vi "EtherCAT Control Simplified interface.vi"() -> ()   [LabVIEW 2022 SP3]
uses:
  MOTION/TypeDefs/EL72xx_DMCOutputs.ctl
  MOTION/TypeDefs/EL72xx_DMCInputs.ctl
  SAFETY/TypeDefs/DeviceInfoData.ctl
  SAFETY/TypeDefs/FSLogicInputs.ctl
  SAFETY/TypeDefs/TwinSAFEGroupInfoData.ctl
  SAFETY/TypeDefs/TwinSAFETerminal.ctl
  IO/TypeDefs/EL2008Outputs.ctl
  <userlib>/Beckhoff-LabVIEW-Interface/_DependsOn/Base/Read/Read Sync.vi
  <userlib>/Beckhoff-LabVIEW-Interface/_DependsOn/Base/TypeResolver/Get TypeResolver.vi
  MOTION/Motion_Library.lvlib
  ADS/ADS_Library.lvlib
  SAFETY/Safety_Library.lvlib
  IO/IO_Library.lvlib
panel:
  in  "stop":bool
  in  "EtherCAT Control":T1(tab)
  in  "Move!":bool
  in  "Motion":string="<PortInfo><Inputs><SymbolControlItems><SymbolControlItem GroupName=\"ADS Write\" GroupDescription=\"Parameters for ADS Write command\"><Parameters><Parameter Name=\"Name\">Term 21 (EL7201-9014).DMC Outputs 32 Bit</Parameter><Parameter Name=\"SymbolName\">Term 21 (EL7201-9014).DMC Outputs 32 Bit</Parameter><Parameter Name=\"SymbolType\">DMC Outputs 32 Bit_1_TYPE</Parameter><Parameter Name=\"SymbolGuid\"></Parameter><Parameter Name=\"AmsNetId\">10.97.0.23.1.1</Parameter><Parameter Name=\"Port\">27911</Parameter><Parameter Name=\"IndexGroup\">#x0</Parameter><Parameter Name=\"IndexOffset\">#x0</Parameter><Parameter Name=\"BitSize\">320</Parameter><Parameter Name=\"CycleTime [ms]\">10</Parameter><Parameter Name=\"Timeout [ms]\">1000</Parameter></Parameters></SymbolControlItem></SymbolControlItems></Inputs><Outputs><SymbolControlItems><SymbolControlItem GroupName=\"ADS Read\" GroupDescription=\"Parameters for ADS Read command\"><Parameters><Parameter Name=\"Name\">Term 21 (EL7201-9014).DMC Inputs 32 Bit</Parameter><Parameter Name=\"SymbolName\">Term 21 (EL7201-9014).DMC Inputs 32 Bit</Parameter><Parameter Name=\"SymbolType\">DMC Inputs 32 Bit_1_TYPE</Parameter><Parameter Name=\"SymbolGuid\"></Parameter><Parameter Name=\"AmsNetId\">10.97.0.23.1.1</Parameter><Parameter Name=\"Port\">27911</Parameter><Parameter Name=\"IndexGroup\">#x0</Parameter><Parameter Name=\"IndexOffset\">#x0</Parameter><Parameter Name=\"BitSize\">512</Parameter><Parameter Name=\"CycleTime [ms]\">10</Parameter><Parameter Name=\"Transmode\">3</Parameter><Parameter Name=\"Timeout [ms]\">1000</Parameter><Parameter Name=\"TCBufferSize [Samples]\">10</Parameter><Parameter Name=\"LVBufferSize [Samples]\">50</Parameter><Parameter Name=\"Expected min delay [ms]\">500</Parameter></Parameters></SymbolControlItem></SymbolControlItems></Outputs></PortInfo>"
  out "bHasMatched":bool
  out "Write Status":bool
  in  "DMC Outputs":T2={"DMC"={"FeedbackControl"={"Enable latch extern on positive edge"=FALSE, "Set counter"=FALSE, "Enable latch extern on negative edge"=FALSE}, "DriveControl"={"Enable"=TRUE, "Reset"=FALSE}, "PositioningControl"={"Execute"=TRUE, "Emergency stop"=FALSE}, "Set counter value"=0, "Target position"=0, "Target velocity"=1000, "Start type"=1, "Target acceleration"=10000, "Target deceleration"=10000}}
  out "data":T3
  out "Read status?":bool
  out "error out":errorcluster
  in  "Error Ackn":bool
  out "Read status?":bool[](array[boolean])
  out "error out 2":errorcluster
  out "output cluster 3":cluster{"SymbolName":string, "Cluster":T4} {"Cluster"."Project CRC" format="%x"}
  out "output cluster 4":cluster{"SymbolName":string, "FSLogic":T5}
  out "output cluster 5":T7
  out "EL1904":T8
  out "EL2904":T8
  in  "TwinSAFE Project":string="<PortInfo><Inputs><SymbolControlItems /></Inputs><Outputs><SymbolControlItems><SymbolControlItem GroupName=\"ADS Read\" GroupDescription=\"Parameters for ADS Read command\"><Parameters><Parameter Name=\"Name\">Term 13 (EL6910).Connection Info Data</Parameter><Parameter Name=\"SymbolName\">Term 13 (EL6910).Connection Info Data</Parameter><Parameter Name=\"SymbolType\">Connection Info Data_1_TYPE</Parameter><Parameter Name=\"SymbolGuid\"></Parameter><Parameter Name=\"AmsNetId\">10.97.0.23.1.1</Parameter><Parameter Name=\"Port\">27911</Parameter><Parameter Name=\"IndexGroup\">#x0</Parameter><Parameter Name=\"IndexOffset\">#x0</Parameter><Parameter Name=\"BitSize\">48</Parameter><Parameter Name=\"CycleTime [ms]\">10</Parameter><Parameter Name=\"Transmode\">3</Parameter><Parameter Name=\"Timeout [ms]\">1000</Parameter><Parameter Name=\"TCBufferSize [Samples]\">10</Parameter><Parameter Name=\"LVBufferSize [Samples]\">50</Parameter><Parameter Name=\"Expected min delay [ms]\">500</Parameter></Parameters></SymbolControlItem><SymbolControlItem GroupName=\"ADS Read\" GroupDescription=\"Parameters for ADS Read command\"><Parameters><Parameter Name=\"Name\">Term 13 (EL6910).Device Info Data</Parameter><Parameter Name=\"SymbolName\">Term 13 (EL6910).Device Info Data</Parameter><Parameter Name=\"SymbolType\">Device Info Data_1_TYPE</Parameter><Parameter Name=\"SymbolGuid\"></Parameter><Parameter Name=\"AmsNetId\">10.97.0.23.1.1</Parameter><Parameter Name=\"Port\">27911</Parameter><Parameter Name=\"IndexGroup\">#x0</Parameter><Parameter Name=\"IndexOffset\">#x0</Parameter><Parameter Name=\"BitSize\">48</Parameter><Parameter Name=\"CycleTime [ms]\">10</Parameter><Parameter Name=\"Transmode\">3</Parameter><Parameter Name=\"Timeout [ms]\">1000</Parameter><Parameter Name=\"TCBufferSize [Samples]\">10</Parameter><Parameter Name=\"LVBufferSize [Samples]\">50</Parameter><Parameter Name=\"Expected min delay [ms]\">500</Parameter></Parameters></SymbolControlItem><SymbolControlItem GroupName=\"ADS Read\" GroupDescription=\"Parameters for ADS Read command\"><Parameters><Parameter Name=\"Name\">Term 13 (EL6910).FSLOGIC Inputs</Parameter><Parameter Name=\"SymbolName\">Term 13 (EL6910).FSLOGIC Inputs</Parameter><Parameter Name=\"SymbolType\">FSLOGIC Inputs_1_TYPE</Parameter><Parameter Name=\"SymbolGuid\"></Parameter><Parameter Name=\"AmsNetId\">10.97.0.23.1.1</Parameter><Parameter Name=\"Port\">27911</Parameter><Parameter Name=\"IndexGroup\">#x0</Parameter><Parameter Name=\"IndexOffset\">#x0</Parameter><Parameter Name=\"BitSize\">16</Parameter><Parameter Name=\"CycleTime [ms]\">10</Parameter><Parameter Name=\"Transmode\">3</Parameter><Parameter Name=\"Timeout [ms]\">1000</Parameter><Parameter Name=\"TCBufferSize [Samples]\">10</Parameter><Parameter Name=\"LVBufferSize [Samples]\">50</Parameter><Parameter Name=\"Expected min delay [ms]\">500</Parameter></Parameters></SymbolControlItem><SymbolControlItem GroupName=\"ADS Read\" GroupDescription=\"Parameters for ADS Read command\"><Parameters><Parameter Name=\"Name\">Term 13 (EL6910).TwinSAFE Group Info Data.TwinSafeGroup1 Info Data</Parameter><Parameter Name=\"SymbolName\">Term 13 (EL6910).TwinSAFE Group Info Data.TwinSafeGroup1 Info Data</Parameter><Parameter Name=\"SymbolType\">INFODATA_GRP_3</Parameter><Parameter Name=\"SymbolGuid\"></Parameter><Parameter Name=\"AmsNetId\">10.97.0.23.1.1</Parameter><Parameter Name=\"Port\">27911</Parameter><Parameter Name=\"IndexGroup\">#x0</Parameter><Parameter Name=\"IndexOffset\">#x0</Parameter><Parameter Name=\"BitSize\">16</Parameter><Parameter Name=\"CycleTime [ms]\">10</Parameter><Parameter Name=\"Transmode\">3</Parameter><Parameter Name=\"Timeout [ms]\">1000</Parameter><Parameter Name=\"TCBufferSize [Samples]\">10</Parameter><Parameter Name=\"LVBufferSize [Samples]\">50</Parameter><Parameter Name=\"Expected min delay [ms]\">500</Parameter></Parameters></SymbolControlItem></SymbolControlItems></Outputs></PortInfo>"
  in  "PLC Safety Control":string="<PortInfo><Inputs><SymbolControlItems><SymbolControlItem GroupName=\"ADS Write\" GroupDescription=\"Parameters for ADS Write command\"><Parameters><Parameter Name=\"Name\">MAIN.SafetyErrAck</Parameter><Parameter Name=\"SymbolName\">MAIN.SafetyErrAck</Parameter><Parameter Name=\"SymbolType\">BOOL</Parameter><Parameter Name=\"SymbolGuid\"></Parameter><Parameter Name=\"AmsNetId\">10.97.0.23.1.1</Parameter><Parameter Name=\"Port\">851</Parameter><Parameter Name=\"IndexGroup\">#x0</Parameter><Parameter Name=\"IndexOffset\">#x0</Parameter><Parameter Name=\"BitSize\">8</Parameter><Parameter Name=\"CycleTime [ms]\">10</Parameter><Parameter Name=\"Timeout [ms]\">1000</Parameter></Parameters></SymbolControlItem></SymbolControlItems></Inputs><Outputs><SymbolControlItems /></Outputs></PortInfo>"
  out "Write Status":bool
  out "bHasMatched":bool
  out "error out 5":errorcluster
  in  "Digital Outputs":string="<PortInfo><Inputs><SymbolControlItems><SymbolControlItem GroupName=\"ADS Write\" GroupDescription=\"Parameters for ADS Write command\"><Parameters><Parameter Name=\"Name\">Term 2 (EL2008).Channel 1.Output</Parameter><Parameter Name=\"SymbolName\">Term 2 (EL2008).Channel 1.Output</Parameter><Parameter Name=\"SymbolType\">BIT</Parameter><Parameter Name=\"SymbolGuid\"></Parameter><Parameter Name=\"AmsNetId\">10.97.0.23.1.1</Parameter><Parameter Name=\"Port\">27905</Parameter><Parameter Name=\"IndexGroup\">#x0</Parameter><Parameter Name=\"IndexOffset\">#x0</Parameter><Parameter Name=\"BitSize\">1</Parameter><Parameter Name=\"CycleTime [ms]\">2</Parameter><Parameter Name=\"Timeout [ms]\">1000</Parameter></Parameters></SymbolControlItem><SymbolControlItem GroupName=\"ADS Write\" GroupDescription=\"Parameters for ADS Write command\"><Parameters><Parameter Name=\"Name\">Term 2 (EL2008).Channel 2.Output</Parameter><Parameter Name=\"SymbolName\">Term 2 (EL2008).Channel 2.Output</Parameter><Parameter Name=\"SymbolType\">BIT</Parameter><Parameter Name=\"SymbolGuid\"></Parameter><Parameter Name=\"AmsNetId\">10.97.0.23.1.1</Parameter><Parameter Name=\"Port\">27905</Parameter><Parameter Name=\"IndexGroup\">#x0</Parameter><Parameter Name=\"IndexOffset\">#x0</Parameter><Parameter Name=\"BitSize\">1</Parameter><Parameter Name=\"CycleTime [ms]\">2</Parameter><Parameter Name=\"Timeout [ms]\">1000</Parameter></Parameters></SymbolControlItem><SymbolControlItem GroupName=\"ADS Write\" GroupDescription=\"Parameters for ADS Write command\"><Parameters><Parameter Name=\"Name\">Term 2 (EL2008).Channel 3.Output</Parameter><Parameter Name=\"SymbolName\">Term 2 (EL2008).Channel 3.Output</Parameter><Parameter Name=\"SymbolType\">BIT</Parameter><Parameter Name=\"SymbolGuid\"></Parameter><Parameter Name=\"AmsNetId\">10.97.0.23.1.1</Parameter><Parameter Name=\"Port\">27905</Parameter><Parameter Name=\"IndexGroup\">#x0</Parameter><Parameter Name=\"IndexOffset\">#x0</Parameter><Parameter Name=\"BitSize\">1</Parameter><Parameter Name=\"CycleTime [ms]\">2</Parameter><Parameter Name=\"Timeout [ms]\">1000</Parameter></Parameters></SymbolControlItem><SymbolControlItem GroupName=\"ADS Write\" GroupDescription=\"Parameters for ADS Write command\"><Parameters><Parameter Name=\"Name\">Term 2 (EL2008).Channel 4.Output</Parameter><Parameter Name=\"SymbolName\">Term 2 (EL2008).Channel 4.Output</Parameter><Parameter Name=\"SymbolType\">BIT</Parameter><Parameter Name=\"SymbolGuid\"></Parameter><Parameter Name=\"AmsNetId\">10.97.0.23.1.1</Parameter><Parameter Name=\"Port\">27905</Parameter><Parameter Name=\"IndexGroup\">#x0</Parameter><Parameter Name=\"IndexOffset\">#x0</Parameter><Parameter Name=\"BitSize\">1</Parameter><Parameter Name=\"CycleTime [ms]\">2</Parameter><Parameter Name=\"Timeout [ms]\">1000</Parameter></Parameters></SymbolControlItem><SymbolControlItem GroupName=\"ADS Write\" GroupDescription=\"Parameters for ADS Write command\"><Parameters><Parameter Name=\"Name\">Term 2 (EL2008).Channel 5.Output</Parameter><Parameter Name=\"SymbolName\">Term 2 (EL2008).Channel 5.Output</Parameter><Parameter Name=\"SymbolType\">BIT</Parameter><Parameter Name=\"SymbolGuid\"></Parameter><Parameter Name=\"AmsNetId\">10.97.0.23.1.1</Parameter><Parameter Name=\"Port\">27905</Parameter><Parameter Name=\"IndexGroup\">#x0</Parameter><Parameter Name=\"IndexOffset\">#x0</Parameter><Parameter Name=\"BitSize\">1</Parameter><Parameter Name=\"CycleTime [ms]\">2</Parameter><Parameter Name=\"Timeout [ms]\">1000</Parameter></Parameters></SymbolControlItem><SymbolControlItem GroupName=\"ADS Write\" GroupDescription=\"Parameters for ADS Write command\"><Parameters><Parameter Name=\"Name\">Term 2 (EL2008).Channel 6.Output</Parameter><Parameter Name=\"SymbolName\">Term 2 (EL2008).Channel 6.Output</Parameter><Parameter Name=\"SymbolType\">BIT</Parameter><Parameter Name=\"SymbolGuid\"></Parameter><Parameter Name=\"AmsNetId\">10.97.0.23.1.1</Parameter><Parameter Name=\"Port\">27905</Parameter><Parameter Name=\"IndexGroup\">#x0</Parameter><Parameter Name=\"IndexOffset\">#x0</Parameter><Parameter Name=\"BitSize\">1</Parameter><Parameter Name=\"CycleTime [ms]\">2</Parameter><Parameter Name=\"Timeout [ms]\">1000</Parameter></Parameters></SymbolControlItem><SymbolControlItem GroupName=\"ADS Write\" GroupDescription=\"Parameters for ADS Write command\"><Parameters><Parameter Name=\"Name\">Term 2 (EL2008).Channel 7.Output</Parameter><Parameter Name=\"SymbolName\">Term 2 (EL2008).Channel 7.Output</Parameter><Parameter Name=\"SymbolType\">BIT</Parameter><Parameter Name=\"SymbolGuid\"></Parameter><Parameter Name=\"AmsNetId\">10.97.0.23.1.1</Parameter><Parameter Name=\"Port\">27905</Parameter><Parameter Name=\"IndexGroup\">#x0</Parameter><Parameter Name=\"IndexOffset\">#x0</Parameter><Parameter Name=\"BitSize\">1</Parameter><Parameter Name=\"CycleTime [ms]\">2</Parameter><Parameter Name=\"Timeout [ms]\">1000</Parameter></Parameters></SymbolControlItem><SymbolControlItem GroupName=\"ADS Write\" GroupDescription=\"Parameters for ADS Write command\"><Parameters><Parameter Name=\"Name\">Term 2 (EL2008).Channel 8.Output</Parameter><Parameter Name=\"SymbolName\">Term 2 (EL2008).Channel 8.Output</Parameter><Parameter Name=\"SymbolType\">BIT</Parameter><Parameter Name=\"SymbolGuid\"></Parameter><Parameter Name=\"AmsNetId\">10.97.0.23.1.1</Parameter><Parameter Name=\"Port\">27905</Parameter><Parameter Name=\"IndexGroup\">#x0</Parameter><Parameter Name=\"IndexOffset\">#x0</Parameter><Parameter Name=\"BitSize\">1</Parameter><Parameter Name=\"CycleTime [ms]\">2</Parameter><Parameter Name=\"Timeout [ms]\">1000</Parameter></Parameters></SymbolControlItem></SymbolControlItems></Inputs><Outputs><SymbolControlItems /></Outputs></PortInfo>"
  out "bHasMatched":bool[](array[boolean])
  out "Write Status":bool[](array[boolean])
  in  "EL2008 Channels":T9
  out "error out 3":errorcluster
  in  "Digital Outputs":string="<PortInfo><Inputs><SymbolControlItems><SymbolControlItem GroupName=\"ADS Write\" GroupDescription=\"Parameters for ADS Write command\"><Parameters><Parameter Name=\"Name\">Box 17 (NI 9145).Module 1 (NI 9472).Digital Output.DO</Parameter><Parameter Name=\"SymbolName\">Box 17 (NI 9145).Module 1 (NI 9472).Digital Output.DO</Parameter><Parameter Name=\"SymbolType\">USINT</Parameter><Parameter Name=\"SymbolGuid\"></Parameter><Parameter Name=\"AmsNetId\">10.97.0.23.1.1</Parameter><Parameter Name=\"Port\">27911</Parameter><Parameter Name=\"IndexGroup\">#x0</Parameter><Parameter Name=\"IndexOffset\">#x0</Parameter><Parameter Name=\"BitSize\">8</Parameter><Parameter Name=\"CycleTime [ms]\">10</Parameter><Parameter Name=\"Timeout [ms]\">1000</Parameter></Parameters></SymbolControlItem></SymbolControlItems></Inputs><Outputs><SymbolControlItems /></Outputs></PortInfo>"
  out "error out":errorcluster
  out "bHasMatched":bool
  out "Write Status":bool
  in  "NI9472":T9
  out "Waveform Chart 2":dbl(graph)
  out "RData":variant
  out "RDataArray":variant[](array[variant])
  out "Read status? 3":bool
  in  "String":string="<PortInfo><Inputs><SymbolControlItems /></Inputs><Outputs><SymbolControlItems><SymbolControlItem GroupName=\"ADS Read\" GroupDescription=\"Parameters for ADS Read command\"><Parameters><Parameter Name=\"Name\">Term 15 (EL3255).AI Standard Channel 1.Value</Parameter><Parameter Name=\"SymbolName\">Term 15 (EL3255).AI Standard Channel 1.Value</Parameter><Parameter Name=\"SymbolType\">INT</Parameter><Parameter Name=\"SymbolGuid\"></Parameter><Parameter Name=\"AmsNetId\">10.97.0.23.1.1</Parameter><Parameter Name=\"Port\">27911</Parameter><Parameter Name=\"IndexGroup\">#x0</Parameter><Parameter Name=\"IndexOffset\">#x0</Parameter><Parameter Name=\"BitSize\">16</Parameter><Parameter Name=\"CycleTime [ms]\">10</Parameter><Parameter Name=\"Transmode\">3</Parameter><Parameter Name=\"Timeout [ms]\">1000</Parameter><Parameter Name=\"TCBufferSize [Samples]\">10</Parameter><Parameter Name=\"LVBufferSize [Samples]\">50</Parameter><Parameter Name=\"Expected min delay [ms]\">500</Parameter></Parameters></SymbolControlItem></SymbolControlItems></Outputs></PortInfo>"
  out "error out 4":errorcluster
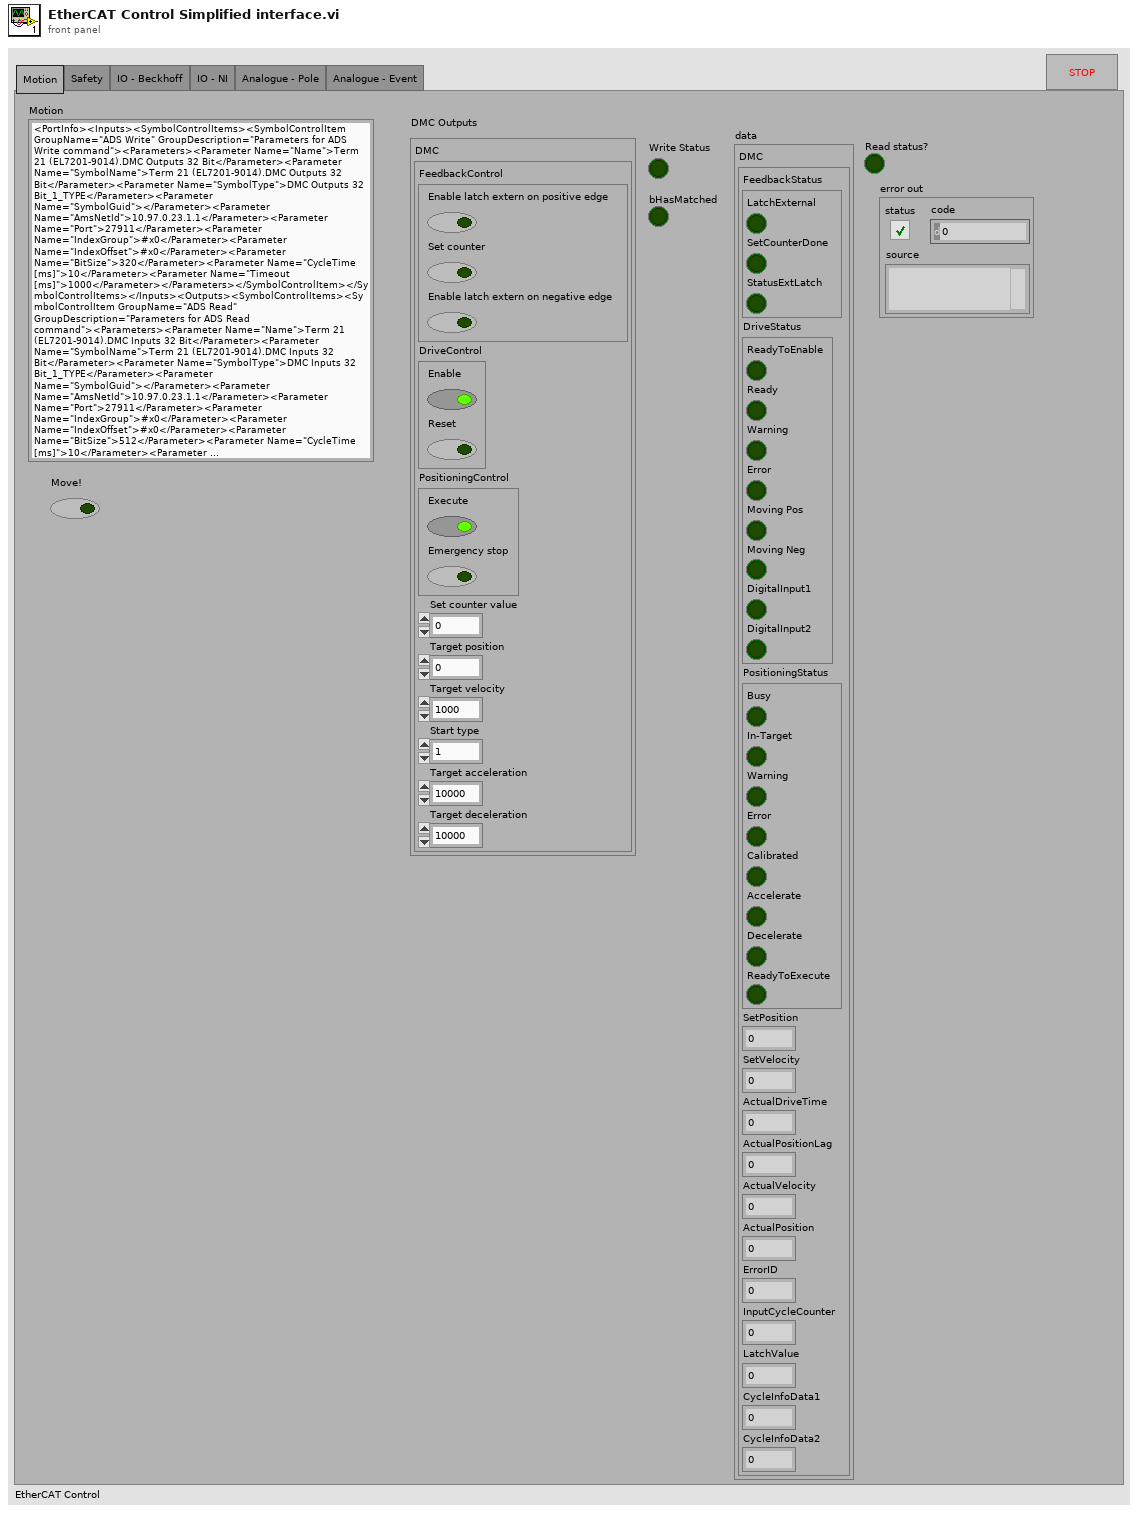
[diagram p1: front panel]
types:
  T1 = enum32{"Motion", "Safety", "IO - Beckhoff", "IO - NI", "Analogue - Pole", "Analogue - Event"}
  T2 = typedef "Motion_Library.lvlib/EL72xx_DMCOutputs.ctl" = cluster{"DMC":cluster{"FeedbackControl":cluster{"Enable latch extern on positive edge":bool, "Set counter":bool, "Enable latch extern on negative edge":bool}, "DriveControl":cluster{"Enable":bool, "Reset":bool}, "PositioningControl":cluster{"Execute":bool, "Emergency stop":bool}, "Set counter value":i32, "Target position":i32, "Target velocity":i16, "Start type":u16, "Target acceleration":u16, "Target deceleration":u16}}
  T3 = typedef "Motion_Library.lvlib/EL72xx_DMCInputs.ctl" = cluster{"DMC":cluster{"FeedbackStatus":cluster{"LatchExternal":bool, "SetCounterDone":bool, "StatusExtLatch":bool}, "DriveStatus":cluster{"ReadyToEnable":bool, "Ready":bool, "Warning":bool, "Error":bool, "Moving Pos":bool, "Moving Neg":bool, "DigitalInput1":bool, "DigitalInput2":bool}, "PositioningStatus":cluster{"Busy":bool, "In-Target":bool, "Warning":bool, "Error":bool, "Calibrated":bool, "Accelerate":bool, "Decelerate":bool, "ReadyToExecute":bool}, "SetPosition":dbl, "SetVelocity":dbl, "ActualDriveTime":dbl, "ActualPositionLag":dbl, "ActualVelocity":dbl, "ActualPosition":dbl, "ErrorID":dbl, "InputCycleCounter":dbl, "LatchValue":dbl, "CycleInfoData1":dbl, "CycleInfoData2":dbl}}
  T4 = typedef "Safety_Library.lvlib/DeviceInfoData.ctl" = cluster{"Project CRC":u16, "Serial Number":u32}
  T5 = typedef "Safety_Library.lvlib/FSLogicInputs.ctl" = cluster{"Safe Logic State":u8, "Cycle Counter":u8}
  T6 = typedef "Safety_Library.lvlib/TwinSAFEGroupInfoData.ctl" = cluster{"State":u8, "Diag":u8}
  T7 = cluster{"SymbolName":string, "Group Info Data":T6}
  T8 = typedef "Safety_Library.lvlib/TwinSAFETerminal.ctl" = cluster{"SymbolName":string, "State":dbl, "Diag":dbl, "Channel 1":bool, "Channel 2":bool, "Channel 3":bool, "Channel 4":bool}
  T9 = typedef "IO_Library.lvlib/EL2008Outputs.ctl" = cluster{"Channel 1":bool, "Channel 2":bool, "Channel 3":bool, "Channel 4":bool, "Channel 5":bool, "Channel 6":bool, "Channel 7":bool, "Channel 8":bool}
  T10 = cluster{"State":dbl, "State 2":dbl, "State 3":i8}
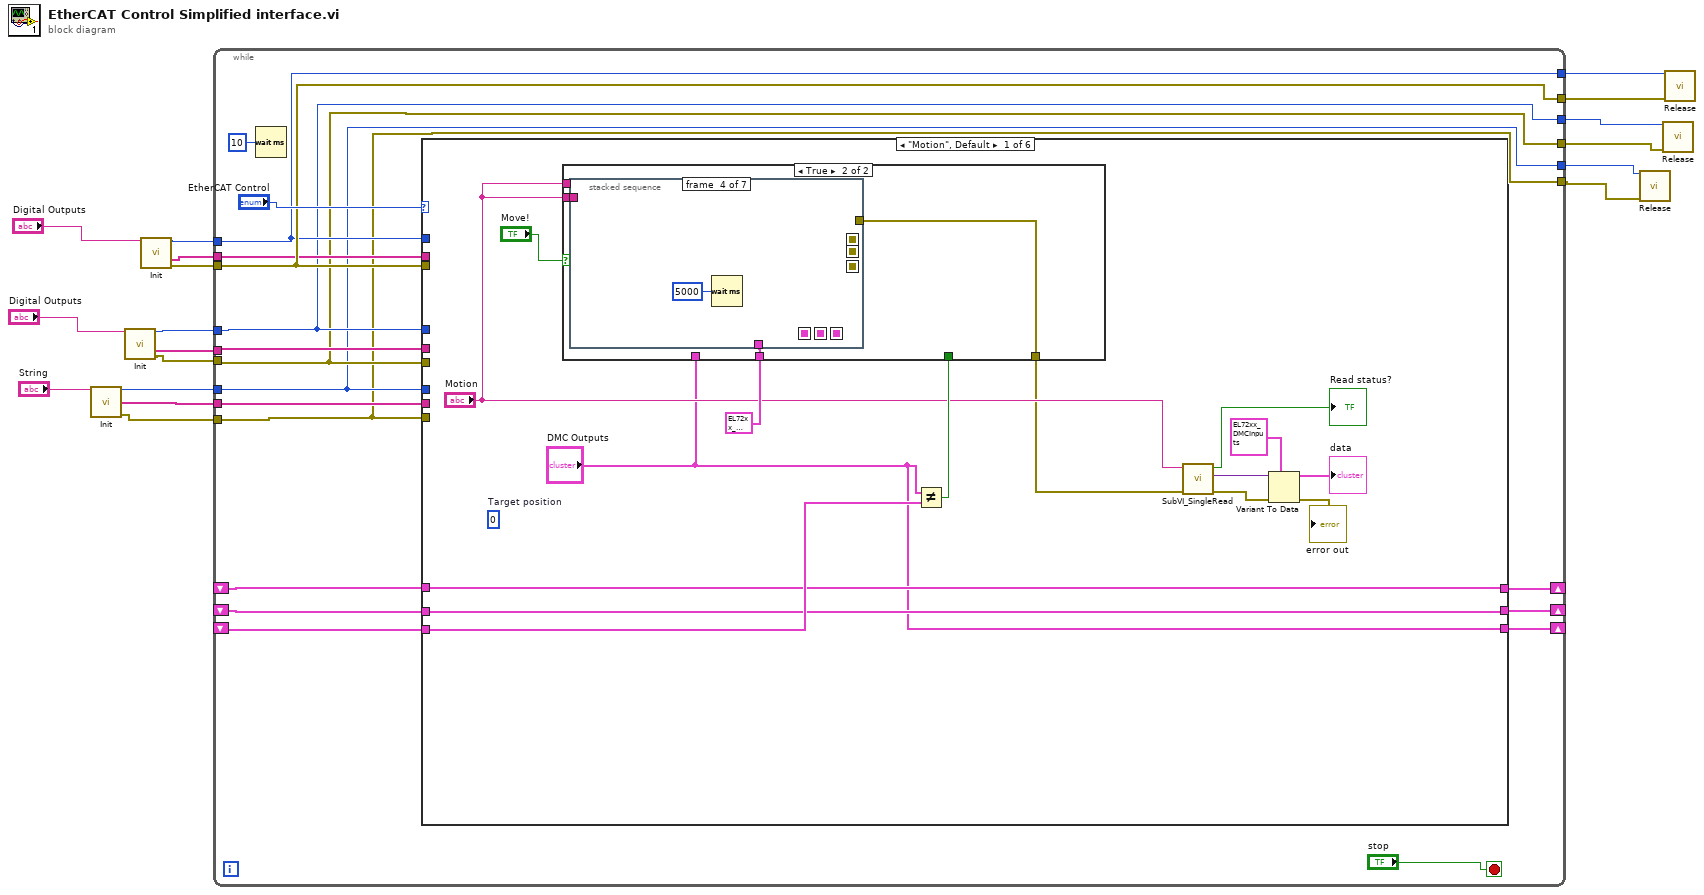
[diagram p0: block diagram]
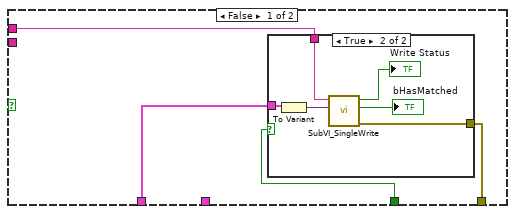
[diagram p2: hidden frame]
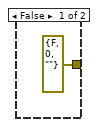
[diagram p3: hidden frame]
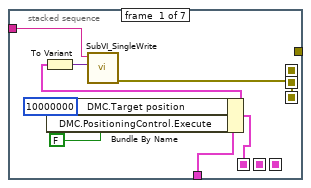
[diagram p4: hidden frame]
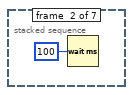
[diagram p5: hidden frame]
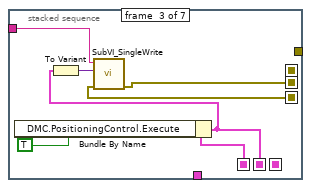
[diagram p6: hidden frame]
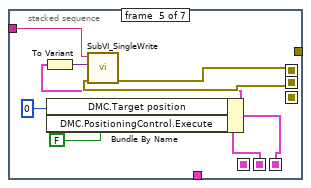
[diagram p7: hidden frame]
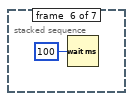
[diagram p8: hidden frame]
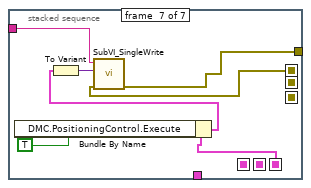
[diagram p9: hidden frame]
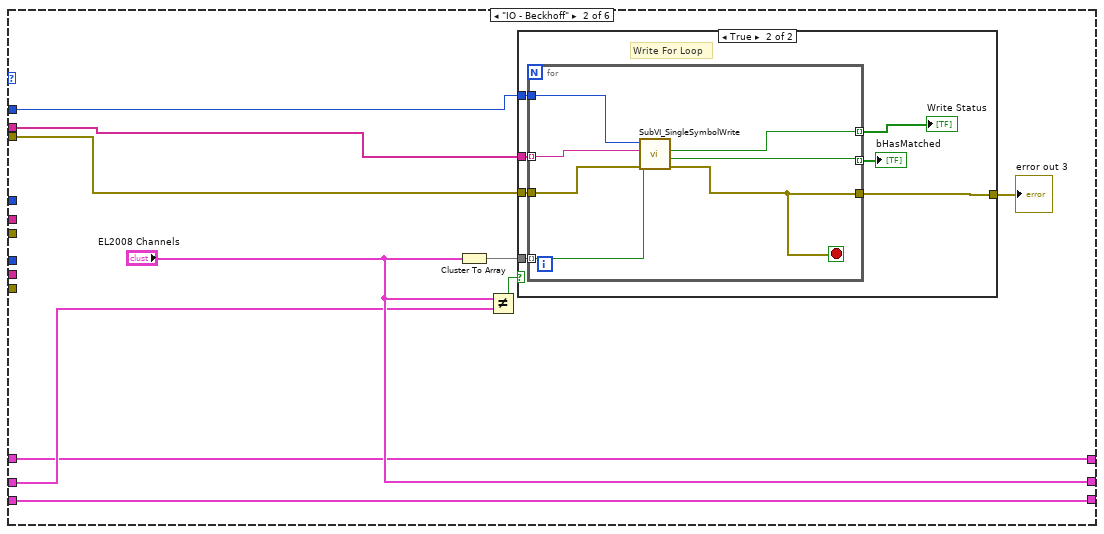
[diagram p10: hidden frame]
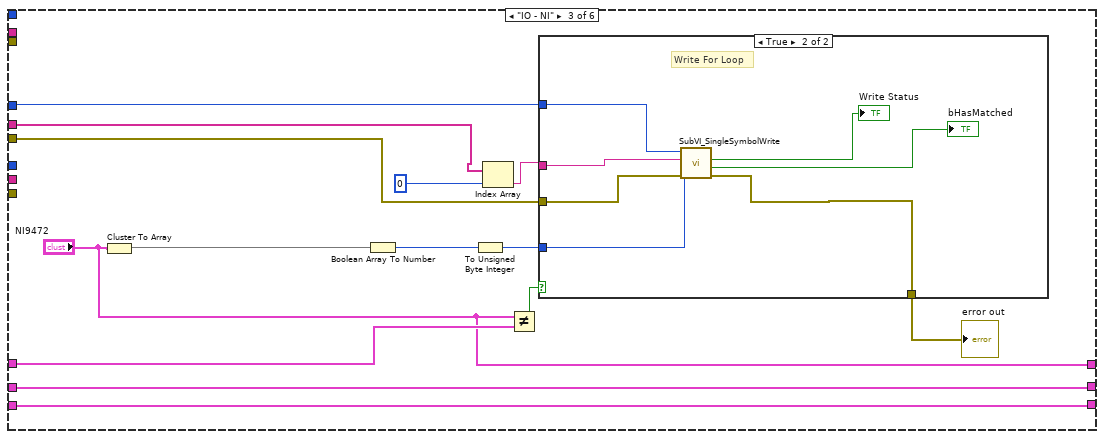
[diagram p12: hidden frame]
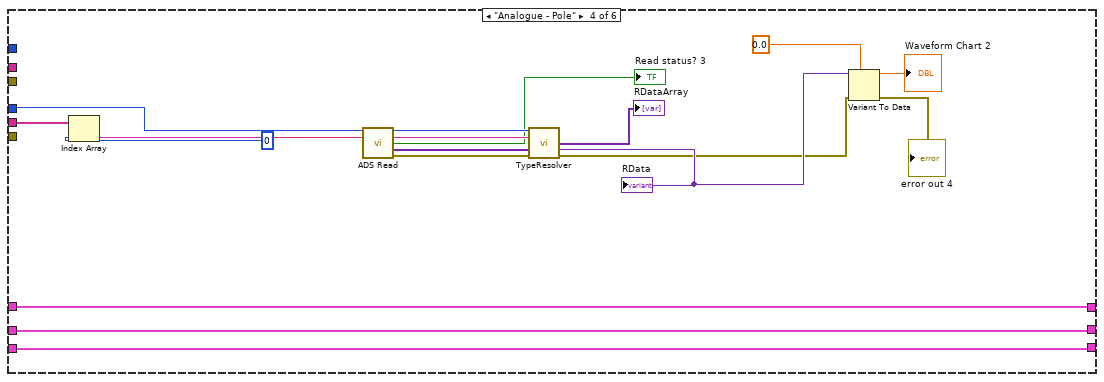
[diagram p14: hidden frame]
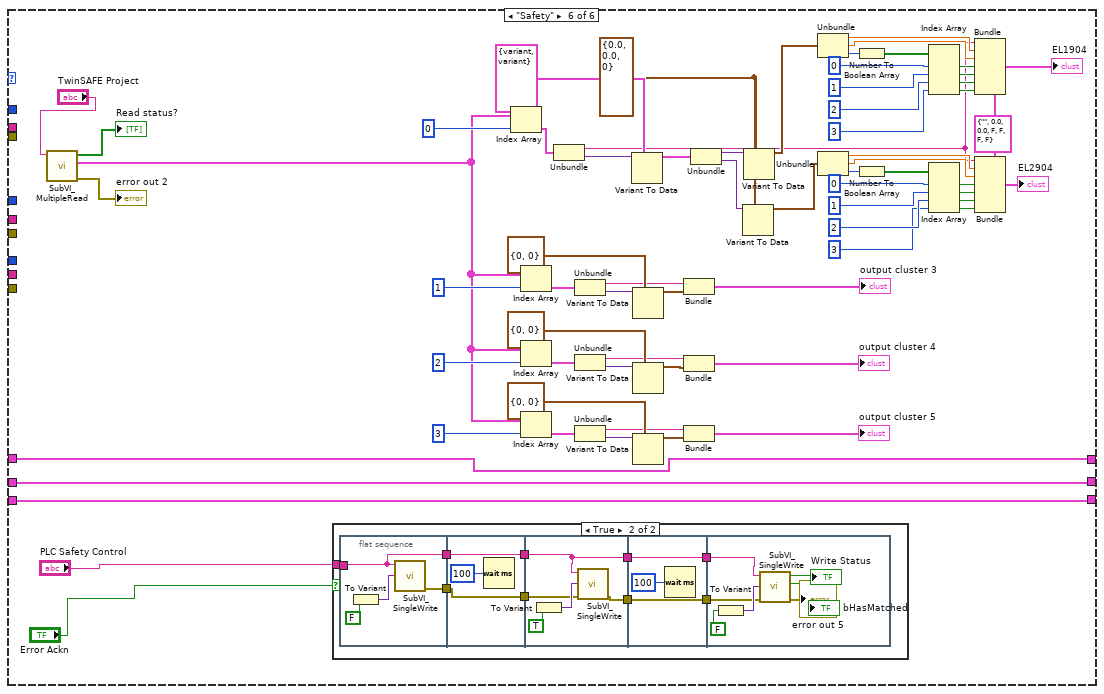
[diagram p16: hidden frame]
diagram:
  n1 = call <userlib>:"Init.vi"("XMLDescription"="String") -> ("Handle"=w5:u32, "ReadGrpSymbols"=w4:string[], "error out"=w3:errorcluster)  [unwired: 10 in, 2 out]
  n2 = call <userlib>:"Init.vi"("XMLDescription"="Digital Outputs") -> ("Handle"=w11:u32, "WriteGrpSymbols"=w10:string[], "error out"=w9:errorcluster)  [unwired: 10 in, 2 out]
  n3 = call <userlib>:"Init.vi"("XMLDescription"="Digital Outputs") -> ("Handle"=w16:u32, "WriteGrpSymbols"=w13:string[], "error out"=w15:errorcluster)  [unwired: 10 in, 2 out]
  n4 = while {
    shift-right: [w32] -> _
    shift-left: _ -> [w33]
    tunnel: [w28] -> w17
    tunnel: w16 -> [w28]
    tunnel: w15 -> [w29]
    tunnel: [w29] -> w14
    shift-right: [w31] -> _
    shift-left: _ -> [w30]
    tunnel: w13 -> [w27]
    tunnel: w11 -> [w25]
    tunnel: w10 -> [w26]
    tunnel: w9 -> [w24]
    tunnel: [w25] -> w8
    tunnel: [w24] -> w7
    shift-right: [w23] -> _
    shift-left: _ -> [w22]
    tunnel: w5 -> [w20]
    tunnel: w4 -> [w21]
    tunnel: w3 -> [w19]
    tunnel: [w20] -> w2
    tunnel: [w19] -> w1
    stop <- "stop" stop-if-true
    n5 = Wait (ms)(milliseconds to wait=u32 10) -> ()  [unwired: 1 out]
    n6 = case shown="\"Motion\", Default" "EtherCAT Control" {
      tunnel: w33 -> [w45 w107 w136 w162 w165 w233]
      tunnel: ["DMC Outputs" w107 w136 w162 w165 w233] -> w32
      tunnel: [w44 "EL2008 Channels" w135 w161 w164 w169] -> w31
      tunnel: w30 -> [w44 w101 w135 w161 w164 w169]
      tunnel: w29 -> [_ w105 _ _ _ _]
      tunnel: w28 -> [_ w104 _ _ _ _]
      tunnel: w27 -> [_ w103 _ _ _ _]
      tunnel: w25 -> [_ _ w134 _ _ _]
      tunnel: w26 -> [_ _ w124 _ _ _]
      tunnel: w24 -> [_ _ w133 _ _ _]
      tunnel: [w43 w98 "NI9472" w160 w163 w168] -> w23
      tunnel: w22 -> [w43 w98 w132 w160 w163 w168]
      tunnel: w20 -> [_ _ _ w146 _ _]
      tunnel: w21 -> [_ _ _ w147 _ _]
      tunnel: w19 -> [_ _ _ _ _ _]
      frame "Motion", Default {
        (unwired) 0  # Target position
        n7 = Not Equal?(x="DMC Outputs", y=w45) -> (x != y?=w40:bool)
        n8 = case shown="True" "Move!" {
          tunnel: "Motion" -> [_ w65]
          tunnel: T2 {"DMC"={"FeedbackControl"={"Enable latch extern on positive edge"=FALSE, "Set counter"=FALSE, "Enable latch extern on negative edge"=FALSE}, "DriveControl"={"Enable"=TRUE, "Reset"=FALSE}, "PositioningControl"={"Execute"=TRUE, "Emergency stop"=FALSE}, "Set counter value"=0, "Target position"=0, "Target velocity"=1000, "Start type"=1, "Target acceleration"=10000, "Target deceleration"=10000}} ("DMC Outputs") -> [_ w64]
          tunnel: w40 -> [w55 _]
          tunnel: "Motion" -> [w54 _]
          tunnel: "DMC Outputs" -> [w53 _]
          tunnel: [w52 w63] -> w37
          frame False {
            n9 = case shown="True" w55 {
              tunnel: w54 -> [_ w62]
              tunnel: [errorcluster {"status"=FALSE, "code"=0, "source"=""} ("error out") w60] -> w52
              tunnel: w53 -> [_ w57]
              frame False {
              }
              frame True {
                n10 = To Variant(anything=w57) -> (Variant=w61:variant)
                n11 = call "SubVI_SingleWrite.vi"("WData"=w61, "String"=w62) -> ("error out"=w60:errorcluster, "bHasMatched"=→"bHasMatched":bool, "Write Status"=→"Write Status":bool)  [unwired: 6 in, 1 out]
              }
            }
          }
          frame True {
            n12 = stacked-sequence {
              seq-local: [w68 _ _ _ _ _ _] -> [_ _ w78 _ _ _ _]
              seq-local: [_ _ w76 _ _ _ _] -> [_ _ _ _ w85 _ _]
              seq-local: [_ _ _ _ w84 _ _] -> [_ _ _ _ _ _ w93]
              seq-local: [w66 _ _ _ _ _ _] -> [_ _ w75 _ _ _ _]
              seq-local: [_ _ w74 _ _ _ _] -> [_ _ _ _ w83 _ _]
              seq-local: [_ _ _ _ w82 _ _] -> [_ _ _ _ _ _ w91]
              tunnel: w65 -> [w67 _ w77 _ w86 _ w94]
              tunnel: w64 -> [w71 _ _ _ _ _ _]
              tunnel: [_ _ _ _ _ _ w92] -> w63
              frame #0 {
                n13 = Bundle By Name(cluster=w71, "DMC.Target position"=10000000, "DMC.PositioningControl.Execute"=FALSE ("DMC.DriveControl.Reset")) -> (w66:T2)
                n14 = To Variant(anything=w66) -> (Variant=w72:variant)
                n15 = call "SubVI_SingleWrite.vi"("WData"=w72, "String"=w67) -> ("error out"=w68:errorcluster)  [unwired: 6 in, 3 out]
              }
              frame #1 {
                n16 = Wait (ms)(milliseconds to wait=u32 100) -> ()  [unwired: 1 out]
              }
              frame #2 {
                n17 = Bundle By Name(cluster=w75, "DMC.PositioningControl.Execute"=TRUE ("DMC.DriveControl.Reset")) -> (w74:T2)
                n18 = To Variant(anything=w74) -> (Variant=w79:variant)
                n19 = call "SubVI_SingleWrite.vi"("error in"=w78, "WData"=w79, "String"=w77) -> ("error out"=w76:errorcluster)  [unwired: 5 in, 3 out]
              }
              frame #3 {
                n20 = Wait (ms)(milliseconds to wait=u32 5000) -> ()  [unwired: 1 out]
              }
              frame #4 {
                n21 = Bundle By Name(cluster=w83, "DMC.Target position"=0, "DMC.PositioningControl.Execute"=FALSE ("DMC.DriveControl.Reset")) -> (w82:T2)
                n22 = To Variant(anything=w82) -> (Variant=w89:variant)
                n23 = call "SubVI_SingleWrite.vi"("error in"=w85, "WData"=w89, "String"=w86) -> ("error out"=w84:errorcluster)  [unwired: 5 in, 3 out]
              }
              frame #5 {
                n24 = Wait (ms)(milliseconds to wait=u32 100) -> ()  [unwired: 1 out]
              }
              frame #6 {
                n25 = Bundle By Name(cluster=w91, "DMC.PositioningControl.Execute"=TRUE ("DMC.DriveControl.Reset")) -> (w95:T2)
                n26 = To Variant(anything=w95) -> (Variant=w96:variant)
                n27 = call "SubVI_SingleWrite.vi"("error in"=w93, "WData"=w96, "String"=w94) -> ("error out"=w92:errorcluster)  [unwired: 5 in, 3 out]
              }
            }
          }
        }
        n28 = call "SubVI_SingleRead.vi"("error in"=w37, "String"="Motion") -> ("error out"=w49:errorcluster, "RData"=w50:variant, "Read status?"=→"Read status?":bool)  [unwired: 6 in]
        n29 = Variant To Data(error in=w49, type=T3 {"DMC"={"FeedbackStatus"={"LatchExternal"=FALSE, "SetCounterDone"=FALSE, "StatusExtLatch"=FALSE}, "DriveStatus"={"ReadyToEnable"=FALSE, "Ready"=FALSE, "Warning"=FALSE, "Error"=FALSE, "Moving Pos"=FALSE, "Moving Neg"=FALSE, "DigitalInput1"=FALSE, "DigitalInput2"=FALSE}, "PositioningStatus"={"Busy"=FALSE, "In-Target"=FALSE, "Warning"=FALSE, "Error"=FALSE, "Calibrated"=FALSE, "Accelerate"=FALSE, "Decelerate"=FALSE, "ReadyToExecute"=FALSE}, "SetPosition"=0.0, "SetVelocity"=0.0, "ActualDriveTime"=0.0, "ActualPositionLag"=0.0, "ActualVelocity"=0.0, "ActualPosition"=0.0, "ErrorID"=0.0, "InputCycleCounter"=0.0, "LatchValue"=0.0, "CycleInfoData1"=0.0, "CycleInfoData2"=0.0}} ("DMC Inputs"), Variant=w50) -> (data=→"data":T3, error out=→"error out":errorcluster)
      }
      frame "IO - Beckhoff" {
        n30 = Cluster To Array(cluster="EL2008 Channels") -> (array=w106:bool[])
        n31 = Not Equal?(x="EL2008 Channels", y=w101) -> (x != y?=w100:bool)
        n32 = case shown="True" w100 {
          tunnel: w106 -> [_ w113]
          tunnel: w105 -> [w108 w112]
          tunnel: w104 -> [_ w111]
          tunnel: w103 -> [_ w110]
          tunnel: [w108 w109] -> w99
          frame False {
          }
          frame True {
            # "Write For Loop"
            n33 = for {
              tunnel: w110 -> [w121] mode=indexing
              tunnel: w112 -> [w120]
              tunnel: w111 -> [w122]
              tunnel: [w118] -> w114 mode=indexing
              tunnel: [w119] -> w115 mode=indexing
              tunnel: w113 -> [w117] mode=indexing
              tunnel: [w116] -> w109
              stop <- w116 stop-if-true
              n34 = call "SubVI_SingleSymbolWrite.vi"("error in"=w120, "WData"=w117, "SymbolName"=w121, "Handle In"=w122) -> ("error out"=w116:errorcluster, "bHasMatched"=w118:bool, "Write Status"=w119:bool)  [unwired: 4 in, 1 out]
            }
            "bHasMatched" <- w114
            "Write Status" <- w115
          }
        }
        "error out 3" <- w99
      }
      frame "IO - NI" {
        n35 = Cluster To Array(cluster="NI9472") -> (array=w129:bool[])
        n36 = Boolean Array To Number(Boolean array=w129) -> (number=w128:u32)
        n37 = To Unsigned Byte Integer(number=w128) -> (unsigned 8bit integer=w127:u8)
        n38 = Index Array(array=w124, index=0) -> (element=w125:string)
        n39 = Not Equal?(x="NI9472", y=w132) -> (x != y?=w131:bool)
        n40 = case shown="True" w131 {
          tunnel: w134 -> [_ w144]
          tunnel: w125 -> [_ w143]
          tunnel: w133 -> [w137 w142]
          tunnel: [w137 w141] -> w130
          tunnel: w127 -> [_ w140]
          frame False {
          }
          frame True {
            # "Write For Loop"
            n41 = call "SubVI_SingleSymbolWrite.vi"("error in"=w142, "WData"=w140, "SymbolName"=w143, "Handle In"=w144) -> ("error out"=w141:errorcluster, "bHasMatched"=→"bHasMatched":bool, "Write Status"=→"Write Status":bool)  [unwired: 4 in, 1 out]
          }
        }
        "error out" <- w130
      }
      frame "Analogue - Pole" {
        n42 = Index Array(array=w147, index=0) -> (element=w158:string)
        n43 = call-poly <userlib>:"ADS Read.vi"("Handle"=w146, "SymbolName"=w158) -> ("Handle"=w157:u32, "SymbolName"=w156:string, "Read status?"=→"Read status? 3":bool, "Ads Read Data"=w155:variant[], "error out"=w154:errorcluster)  [unwired: 9 in]
        n44 = call-poly <userlib>:"TypeResolver.vi"("Handle"=w157, "SymbolName"=w156, "ADSRData"=w155, "error in"=w154) -> ("RDataArray"=→"RDataArray":variant[], "RData"=w152:variant, "error out"=w151:errorcluster)  [unwired: 8 in, 1 out]
        "RData" <- w152
        n45 = Variant To Data(error in=w151, type=0.0, Variant=w152) -> (data=→"Waveform Chart 2":dbl, error out=→"error out 4":errorcluster)
      }
      frame "Analogue - Event" {
      }
      frame "Safety" {
        w172 = T8 {"SymbolName"="", "State"=0.0, "Diag"=0.0, "Channel 1"=FALSE, "Channel 2"=FALSE, "Channel 3"=FALSE, "Channel 4"=FALSE} ("EL1904 2")
        w201 = T10 {"State"=0.0, "State 2"=0.0, "State 3"=0}
        n46 = call "SubVI_MultipleRead.vi"("String"="TwinSAFE Project") -> ("error out"=→"error out 2":errorcluster, "Data"=w226:cluster{"SymbolName":string, "RData":variant}[], "Read status?"=→"Read status?":bool[])  [unwired: 8 in]
        n47 = case shown="True" "Error Ackn" {
          tunnel: "PLC Safety Control" -> [_ w242]
          frame False {
          }
          frame True {
            n48 = flat-sequence {
              tunnel: w242 -> [w244]
              tunnel: [w244] -> w240
              tunnel: [w243] -> w239
              tunnel: [w248] -> w241
              tunnel: w240 -> [w248]
              tunnel: w239 -> [w247]
              tunnel: [w247] -> w238
              tunnel: w241 -> [w251]
              tunnel: w238 -> [w252]
              tunnel: [w251] -> w236
              tunnel: [w250] -> w234
              tunnel: [w257] -> w237
              tunnel: w236 -> [w257]
              tunnel: [w256] -> w235
              tunnel: w234 -> [w256]
              tunnel: w237 -> [w263]
              tunnel: w235 -> [w262]
              frame #0 {
                n49 = To Variant(anything=FALSE ("Error Ack")) -> (Variant=w246:variant)
                n50 = call "SubVI_SingleWrite.vi"("WData"=w246, "String"=w244) -> ("error out"=w243:errorcluster)  [unwired: 6 in, 3 out]
              }
              frame #1 {
                n51 = Wait (ms)(milliseconds to wait=u32 100) -> ()  [unwired: 1 out]
              }
              frame #2 {
                n52 = To Variant(anything=TRUE ("Error Ack")) -> (Variant=w253:variant)
                n53 = call "SubVI_SingleWrite.vi"("error in"=w252, "WData"=w253, "String"=w251) -> ("error out"=w250:errorcluster)  [unwired: 5 in, 3 out]
              }
              frame #3 {
                n54 = Wait (ms)(milliseconds to wait=u32 100) -> ()  [unwired: 1 out]
              }
              frame #4 {
                n55 = To Variant(anything=FALSE ("Error Ack")) -> (Variant=w264:variant)
                n56 = call "SubVI_SingleWrite.vi"("error in"=w262, "WData"=w264, "String"=w263) -> ("error out"=→"error out 5":errorcluster, "bHasMatched"=→"bHasMatched":bool, "Write Status"=→"Write Status":bool)  [unwired: 5 in, 1 out]
              }
            }
          }
        }
        n57 = Index Array(array=w226, index=0) -> (element=w207:cluster{"SymbolName":string, "RData":variant})
        n58 = Index Array(array=w226, index=1) -> (element=w225:cluster{"SymbolName":string, "RData":variant})
        n59 = Index Array(array=w226, index=2) -> (element=w224:cluster{"SymbolName":string, "RData":variant})
        n60 = Index Array(array=w226, index=3) -> (element=w223:cluster{"SymbolName":string, "RData":variant})
        n61 = Unbundle(w207) -> ("SymbolName"=w174:string, "RData"=w206:variant)
        n62 = Unbundle(w225) -> ("SymbolName"=w216:string, "RData"=w220:variant)
        n63 = Unbundle(w224) -> ("SymbolName"=w215:string, "RData"=w221:variant)
        n64 = Unbundle(w223) -> ("SymbolName"=w214:string, "RData"=w222:variant)
        n65 = Variant To Data(type=cluster{variant, variant} {variant, variant}, Variant=w206) -> (data=w204:cluster{variant, variant})  [unwired: 1 in, 1 out]
        n66 = Variant To Data(type=T4 {"Project CRC"=0, "Serial Number"=0} ("Cluster"), Variant=w220) -> (data=w213:T4)  [unwired: 1 in, 1 out]
        n67 = Variant To Data(type=T5 {"Safe Logic State"=0, "Cycle Counter"=0} ("FSLogic"), Variant=w221) -> (data=w212:T5)  [unwired: 1 in, 1 out]
        n68 = Variant To Data(type=T6 {"State"=0, "Diag"=0} ("Group Info Data"), Variant=w222) -> (data=w211:T6)  [unwired: 1 in, 1 out]
        n69 = Bundle("SymbolName"=w216, "Cluster"=w213) -> (→"output cluster 3":cluster{"SymbolName":string, "Cluster":T4})  [unwired: 1 in]
        n70 = Bundle("SymbolName"=w215, "FSLogic"=w212) -> (→"output cluster 4":cluster{"SymbolName":string, "FSLogic":T5})  [unwired: 1 in]
        n71 = Bundle("SymbolName"=w214, "Group Info Data"=w211) -> (→"output cluster 5":T7)  [unwired: 1 in]
        n72 = Unbundle(w204) -> (w203:variant, w202:variant)
        n73 = Variant To Data(type=w201, Variant=w202) -> (data=w176:T10)  [unwired: 1 in, 1 out]
        n74 = Variant To Data(type=w201, Variant=w203) -> (data=w200:T10)  [unwired: 1 in, 1 out]
        n75 = Unbundle(w200) -> ("State"=w192:dbl, "State 2"=w193:dbl, "State 3"=w199:i8)
        n76 = Unbundle(w176) -> ("State"=w181:dbl, "State 2"=w182:dbl, "State 3"=w187:i8)
        n77 = Number To Boolean Array(number=w199) -> (Boolean array=w198:bool[])
        n78 = Number To Boolean Array(number=w187) -> (Boolean array=w186:bool[])
        n79 = Index Array(array=w198, index #1=0 ("index"), index #2=1 ("index"), index #3=2 ("index"), index #4=3 ("index")) -> (element #1=w191:bool, element #2=w190:bool, element #3=w189:bool, element #4=w188:bool)
        n80 = Index Array(array=w186, index #1=0 ("index"), index #2=1 ("index"), index #3=2 ("index"), index #4=3 ("index")) -> (element #1=w180:bool, element #2=w179:bool, element #3=w178:bool, element #4=w177:bool)
        n81 = Bundle(cluster=w172, "SymbolName"=w174, "State"=w192, "Diag"=w193, "Channel 1"=w191, "Channel 2"=w190, "Channel 3"=w189, "Channel 4"=w188) -> (→"EL1904":T8)
        n82 = Bundle(cluster=w172, "SymbolName"=w174, "State"=w181, "Diag"=w182, "Channel 1"=w180, "Channel 2"=w179, "Channel 3"=w178, "Channel 4"=w177) -> (→"EL2904":T8)
      }
    }
  }
  n83 = call <userlib>:"Release.vi"("Handle"=w2, "error in (no error)"=w1) -> ()  [unwired: 13 in, 1 out]
  n84 = call <userlib>:"Release.vi"("Handle"=w8, "error in (no error)"=w7) -> ()  [unwired: 13 in, 1 out]
  n85 = call <userlib>:"Release.vi"("Handle"=w17, "error in (no error)"=w14) -> ()  [unwired: 13 in, 1 out]
